vi "setLaserPower.vi"(4 "error in (no error)":errorcluster, 7 "Power (V)":dbl format="%.2f") -> (0 "error out":errorcluster)   [LabVIEW 2012]
uses:
  bin/OVA32.dll
panel:
  out "DLL Return Code":i32
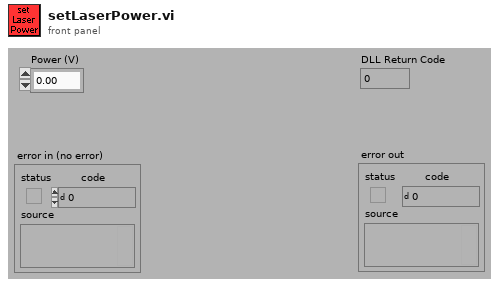
[diagram p1: front panel]
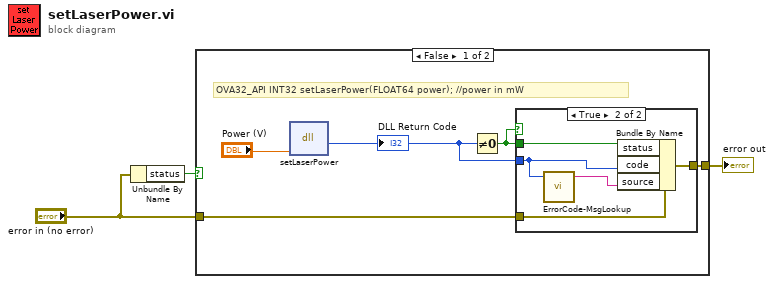
[diagram p0: block diagram]
diagram:
  n1 = Unbundle By Name("error in (no error)") -> ("status"=w2:bool)
  n2 = case shown="False" w2 {
    tunnel: "error in (no error)" -> [w8 w15]
    tunnel: [w7 w15] -> w3
    frame False {
      # "OVA32_API INT32 setLaserPower(FLOAT64 power); //power in mW"
      n3 = dll-call lib="C:/_src/OVA5000_DSP_falcon/Software/LabVIEW/OVA/SDK/OVA_5000_SDK_v5.14.3/bin/OVA32.dll" fn="setLaserPower"("status"="Power (V)") -> (w6:i32)  [unwired: 4 in, 2 out]
      "DLL Return Code" <- w6
      n4 = Not Equal To 0?(x=w6) -> (x != 0?=w5:bool)
      n5 = case shown="True" w5 {
        tunnel: w8 -> [w9 w14]
        tunnel: w5 -> [_ w13]
        tunnel: [w9 w12] -> w7
        tunnel: w6 -> [_ w11]
        frame False {
        }
        frame True {
          n6 = call "ErrorCode-MsgLookup.vi"("DLL Return Code"=w11) -> ("Error String"=w10:string)  [unwired: 2 in, 2 out]
          n7 = Bundle By Name(cluster=w14, "status"=w13, "code"=w11, "source"=w10) -> (w12:errorcluster)
        }
      }
    }
    frame True {
    }
  }
  "error out" <- w3
